vi "MMEM_STOR_TRAC_CONT_CIT.vi"(0 "VISA IN":refnum<visa-resource-name>, 5 "error in":errorcluster, 7 "Format":string(combo)="AUTO") -> (14 "VISA Out":refnum<visa-resource-name>, 19 "error out":errorcluster)   [LabVIEW 2018, in "PNA-X.lvlib"]
doc: "MMEMory:STORe:TRACe:CONTents:CITifile <char> \n(Read-Write) Specifies the contents of subsequent citifile save statements. (See Data Define Saves) \nParameters \n<char> Choose from: \nSING - Single trace \nDISP - All displayed traces \nAUTO - All displayed traces \nExamples MMEM:STOR:TRAC:CONT:CIT SING \nQuery Syntax MMEMory:STORe:TRACe:CONTents? \nReturn Type Character \nDefault Auto"
uses:
  PNA-X.lvlib
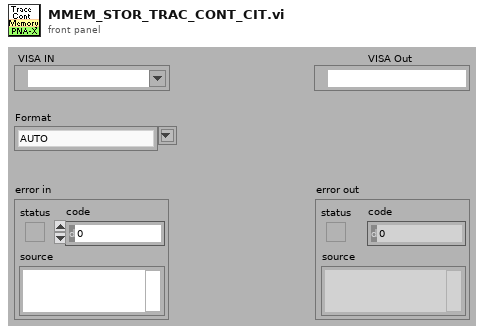
[diagram p1: front panel]
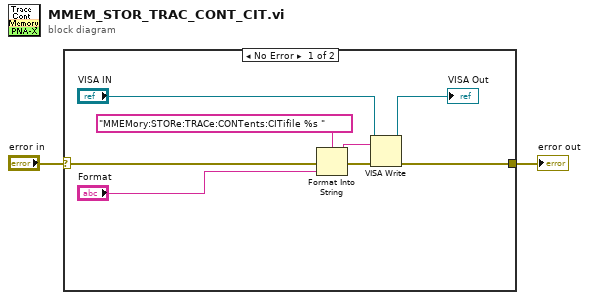
[diagram p0: block diagram]
diagram:
  n1 = case shown="No Error" "error in" {
    selector: "error in" -> [w10 w11]
    tunnel: [w5 w11] -> w1
    frame No Error {
      n2 = Format Into String(format string="MMEMory:STORe:TRACe:CONTents:CITifile %s " ("Cmdline"), error in=w10, "Format") -> (resulting string=w8:string, error out=w9:errorcluster)  [unwired: 1 in]
      n3 = VISA Write(VISA resource name="VISA IN", write buffer=w8, error in (no error)=w9) -> (VISA resource name out=→"VISA Out":refnum<visa-resource-name>, error out=w5:errorcluster)  [unwired: 1 out]
    }
    frame Error {
    }
  }
  "error out" <- w1
